vi "Manipulator Set Dynamics.vi"(8 "error in (no error)":errorcluster, 10 "Inputs":T1, 11 "VISA resource in":refnum<visa-resource-name>="COM1") -> (0 "error out":errorcluster, 2 "Response":T2, 3 "VISA resource out":refnum<visa-resource-name>)   [LabVIEW 2012, in "Scientifica Manipulator Daemon.lvlib"]
uses:
  Scientifica Manipulator Daemon.lvlib
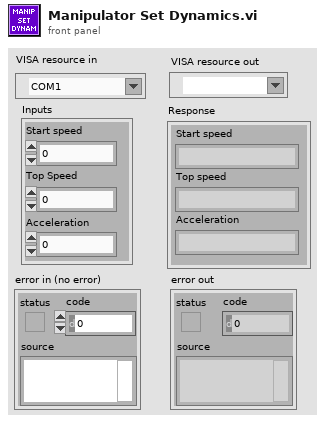
[diagram p1: front panel]
types:
  T1 = cluster{"Start speed":i32, "Top Speed":i32, "Acceleration":i32}
  T2 = cluster{"Start speed":string, "Top speed":string, "Acceleration":string}
  T3 = cluster{"Response":string, "Response":string, "Response":string}
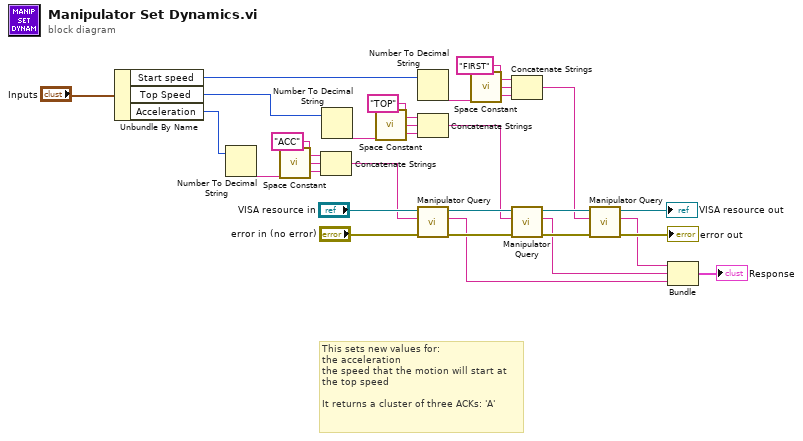
[diagram p0: block diagram]
diagram:
  # "This sets new values for: \nthe acceleration\nthe speed that the motion will start at \nthe top speed\n\nIt returns a cluster of three ACKs: 'A'"
  n1 = Unbundle By Name("Inputs") -> ("Start speed"=w18:i32, "Top Speed"=w19:i32, "Acceleration"=w17:i32)
  n2 = Number To Decimal String(number=w17) -> (decimal integer string=w20:string)  [unwired: 1 in]
  n3 = call <vilib>:"Space Constant.vi"() -> ("String"=w22:string)
  n4 = Concatenate Strings("ACC", w22, w20) -> (w7:string)
  n5 = Number To Decimal String(number=w19) -> (decimal integer string=w23:string)  [unwired: 1 in]
  n6 = call <vilib>:"Space Constant.vi"() -> ("String"=w25:string)
  n7 = Number To Decimal String(number=w18) -> (decimal integer string=w26:string)  [unwired: 1 in]
  n8 = Concatenate Strings("TOP", w25, w23) -> (w6:string)
  n9 = call "Manipulator Query.vi"("error in (no error)"="error in (no error)", "Command"=w7, "VISA resource in"="VISA resource in") -> ("error out"=w9:errorcluster, "Response"=w4:string, "VISA resource out"=w11:refnum<visa-resource-name>)  [unwired: 5 in, 1 out]
  n10 = call <vilib>:"Space Constant.vi"() -> ("String"=w28:string)
  n11 = Concatenate Strings("FIRST", w28, w26) -> (w5:string)
  n12 = call "Manipulator Query.vi"("error in (no error)"=w9, "Command"=w6, "VISA resource in"=w11) -> ("error out"=w8:errorcluster, "Response"=w3:string, "VISA resource out"=w10:refnum<visa-resource-name>)  [unwired: 5 in, 1 out]
  n13 = call "Manipulator Query.vi"("error in (no error)"=w8, "Command"=w5, "VISA resource in"=w10) -> ("error out"=→"error out":errorcluster, "Response"=w2:string, "VISA resource out"=→"VISA resource out":refnum<visa-resource-name>)  [unwired: 5 in, 1 out]
  n14 = Bundle("Response"=w2, "Response"=w3, "Response"=w4) -> (→"Response":T3)  [unwired: 1 in]
